vi "processesAbsorptionImage.vi"(8 "error in (no error)":errorcluster, 9 "FileNeologist.lvclass out":refnum<class "FileNeologist.lvclass">, 10 "ImagePaths in":path[](array[path])) -> (0 "error out":errorcluster, 1 "atomNumber":dbl, 2 "ImagePaths out":path[](array[path]), 3 "BECImageProcessor out":refnum<class "BECImageProcessor.lvclass">, 4 "cloudWidth x":dbl, 5 "cloudWidth z":dbl)   [LabVIEW 2009, in "Tools.lvlib" / "Imaging.lvlib" / "BECImageProcessor.lvclass"]
uses:
  BECImageProcessor.lvclass
  Filing/FileNeologist/FileNeologist.lvclass
  <vilib>/vision/NI_Vision_Development_Module.lvlib
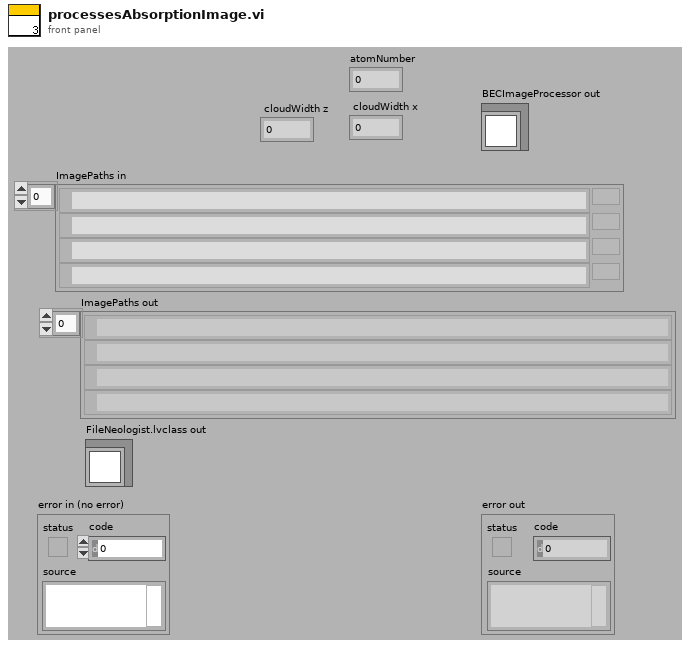
[diagram p1: front panel]
types:
  T1 = typedef "Image Type" = u32
  T2 = typedef "IMAQ Image.ctl" = refnum<image>
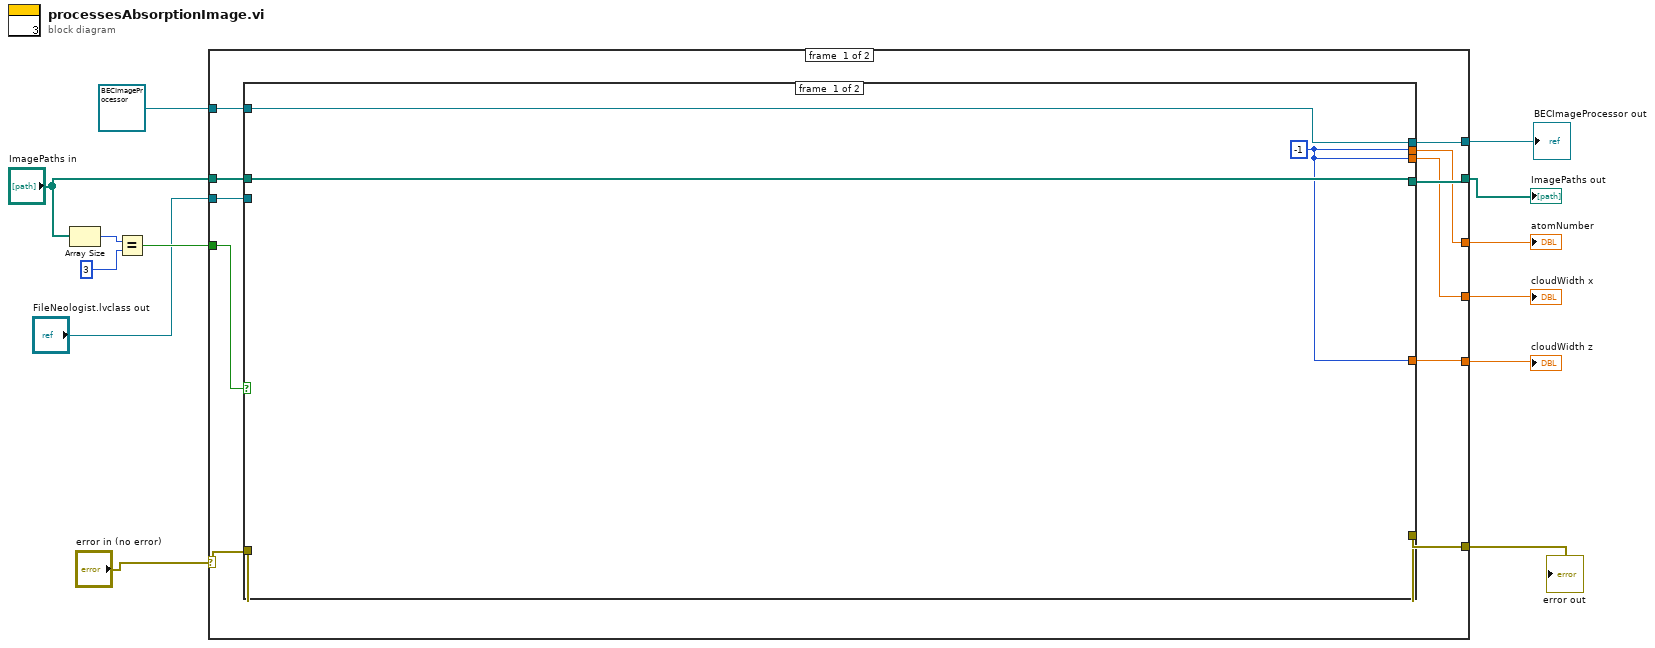
[diagram p0: block diagram]
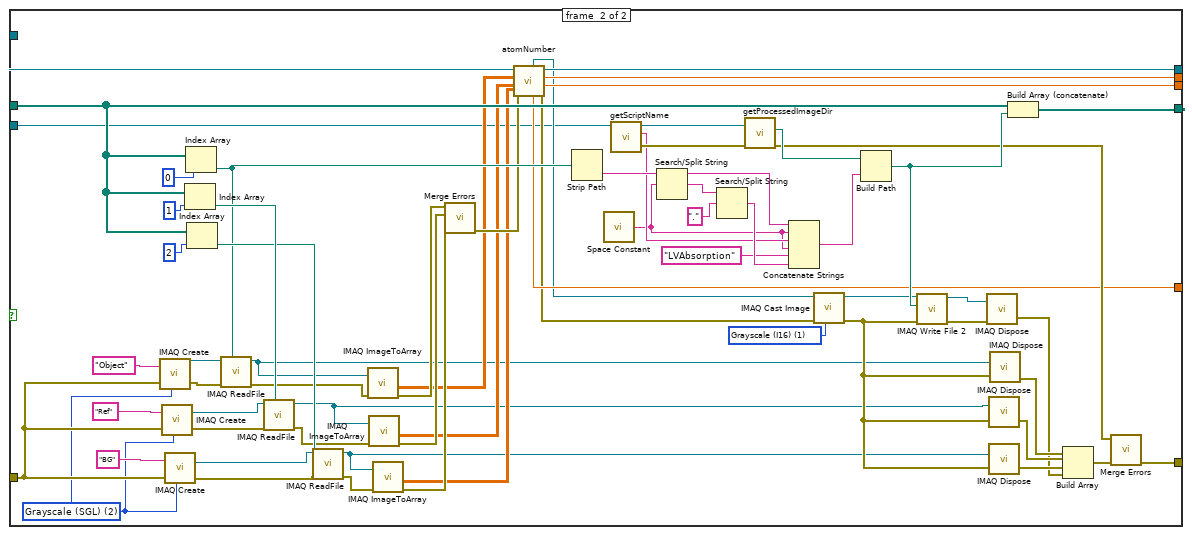
[diagram p2: hidden frame]
diagram:
  n1 = Array Size(array="ImagePaths in") -> (size(s)=w7:i32)
  n2 = Equal?(x=w7, y=3) -> (x = y?=w5:bool)
  n3 = case shown="No Error" "error in (no error)" {
    selector: "error in (no error)" -> [w24 w95]
    tunnel: [w21 w95] -> w10
    tunnel: [w18 w94] -> w12
    tunnel: refnum<class "BECImageProcessor.lvclass"> refnum ("BECImageProcessor in") -> [w19 w94]
    tunnel: "ImagePaths in" -> [w23 _]
    tunnel: [w22 _] -> w11
    tunnel: w5 -> [w20 _]
    tunnel: [w17 _] -> w4
    tunnel: [w16 _] -> w3
    tunnel: [w15 _] -> w2
    tunnel: "FileNeologist.lvclass out" -> [w14 _]
    frame #0 {
      n4 = case shown="True" w20 {
        tunnel: w24 -> [w27 w86]
        tunnel: w23 -> [w28 w78]
        tunnel: [w28 w77] -> w22
        tunnel: [w27 w68] -> w21
        tunnel: w19 -> [w26 w46]
        tunnel: [w26 w41] -> w18
        tunnel: [w25 w40] -> w17
        tunnel: [w25 w39] -> w16
        tunnel: [w25 w38] -> w15
        tunnel: w14 -> [_ w29]
        frame #0 {
          w25 = -1
        }
        frame #1 {
          w60 = T1 1 items=["Grayscale (U8)", "Grayscale (I16)", "Grayscale (SGL)", "Complex (CSG)", "RGB (U32)", "HSL (U32)", "RGB (U64)"] ("Image Type")
          w50 = T1 2 items=["Grayscale (U8)", "Grayscale (I16)", "Grayscale (SGL)", "Complex (CSG)", "RGB (U32)", "HSL (U32)", "RGB (U64)"] ("Image Type")
          n5 = call "IMAQ Create"("Image Name"="Object", "Image Type"=w50, "error in (no error)"=w86) -> ("New Image"=w62:T2, "error out"=w67:errorcluster)  [unwired: 2 in]
          n6 = call "IMAQ Create"("Image Name"="Ref", "Image Type"=w50, "error in (no error)"=w86) -> ("New Image"=w66:T2, "error out"=w65:errorcluster)  [unwired: 2 in]
          n7 = call "IMAQ Create"("Image Name"="BG", "Image Type"=w50, "error in (no error)"=w86) -> ("New Image"=w64:T2, "error out"=w63:errorcluster)  [unwired: 2 in]
          n8 = Index Array(array=w78, index=1) -> (element=w88:path)
          n9 = Index Array(array=w78, index=0) -> (element=w85:path)
          n10 = Index Array(array=w78, index=2) -> (element=w87:path)
          n11 = call "IMAQ ReadFile"("File Path"=w85, "error in (no error)"=w67, "Image"=w62) -> ("error out"=w37:errorcluster, "Image Out"=w34:T2)  [unwired: 4 in, 3 out]
          n12 = call "IMAQ ReadFile"("File Path"=w88, "error in (no error)"=w65, "Image"=w66) -> ("error out"=w36:errorcluster, "Image Out"=w33:T2)  [unwired: 4 in, 3 out]
          n13 = call "IMAQ ReadFile"("File Path"=w87, "error in (no error)"=w63, "Image"=w64) -> ("error out"=w35:errorcluster, "Image Out"=w32:T2)  [unwired: 4 in, 3 out]
          n14 = call "IMAQ ImageToArray"("error in (no error)"=w37, "Image"=w34) -> ("Image Pixels (Float)"=w44:sgl[][], "error out"=w49:errorcluster)  [unwired: 2 in, 3 out]
          n15 = call "IMAQ ImageToArray"("error in (no error)"=w36, "Image"=w33) -> ("Image Pixels (Float)"=w43:sgl[][], "error out"=w48:errorcluster)  [unwired: 2 in, 3 out]
          n16 = call "IMAQ ImageToArray"("error in (no error)"=w35, "Image"=w32) -> ("Image Pixels (Float)"=w42:sgl[][], "error out"=w47:errorcluster)  [unwired: 2 in, 3 out]
          n17 = call <vilib>:"Merge Errors.vi"("error in 3 (no error)"=w47, "error in 2 (no error)"=w48, "error in 1 (no error)"=w49) -> ("error out"=w45:errorcluster)  [unwired: 4 in]
          n18 = call "atomNumber.vi"("Image bg"=w42, "error in (no error)"=w45, "Image ref"=w43, "Image object"=w44, "BECImageProcessor in"=w46) -> ("error out"=w31:errorcluster, "x width"=w39:dbl, "number"=w40:dbl, "BECImageProcessor out"=w41:refnum<class "BECImageProcessor.lvclass">, "z width"=w38:dbl, "Image Out"=w30:T2)  [unwired: 1 in]
          n19 = Strip Path(path=w85) -> (name=w83:string)  [unwired: 1 out]
          n20 = call <vilib>:"Space Constant.vi"() -> ("String"=w51:string)
          n21 = call-dynamic "getScriptName.vi"("FileNeologist.lvclass in"=w29) -> ("error out"=w54:errorcluster, "scriptName"=w53:string, "FileNeologist.lvclass out"=w55:refnum<class "FileNeologist.lvclass">)  [unwired: 8 in]
          n22 = Search/Split String(string=w83, search string/char (-)=w51) -> (substring before match=w81:string, match + rest of string=w82:string)  [unwired: 1 in, 1 out]
          n23 = Search/Split String(string=w82, search string/char (-)=".") -> (match + rest of string=w80:string)  [unwired: 1 in, 2 out]
          n24 = call-dynamic "getProcessedImageDir.vi"("error in (no error)"=w54, "FileNeologist in"=w55) -> ("error out"=w57:errorcluster, "Path"=w58:path)  [unwired: 7 in, 1 out]
          n25 = Concatenate Strings(w81, w51, w53, w51, "LVAbsorption", w80) -> (w79:string)
          n26 = call "IMAQ Cast Image"("Image Type"=w60, "error in (no error)"=w31, "Image Src"=w30) -> ("error out"=w61:errorcluster, "Image Dst Out"=w59:T2)  [unwired: 7 in]
          n27 = Build Path(base path=w58, name or relative path=w79) -> (appended path=w76:path)
          n28 = call-poly "IMAQ Write File 2"("error in (no error)"=w61, "File Path"=w76, "Image"=w59) -> ("error out"=w74:errorcluster, "Image Out (duplicate)"=w75:T2)  [unwired: 7 in]
          n29 = call "IMAQ Dispose"("Image"=w75, "error in (no error)"=w74) -> ("error out"=w70:errorcluster)  [unwired: 4 in]
          n30 = call "IMAQ Dispose"("Image"=w33, "error in (no error)"=w61) -> ("error out"=w72:errorcluster)  [unwired: 4 in]
          n31 = call "IMAQ Dispose"("Image"=w32, "error in (no error)"=w61) -> ("error out"=w71:errorcluster)  [unwired: 4 in]
          n32 = call "IMAQ Dispose"("Image"=w34, "error in (no error)"=w61) -> ("error out"=w73:errorcluster)  [unwired: 4 in]
          n33 = Build Array (concatenate)(w78, w76) -> (w77:path[])
          n34 = Build Array(w73, w72, w71, w70) -> (w69:errorcluster[])
          n35 = call <vilib>:"Merge Errors.vi"("error array in"=w69, "error in 1 (no error)"=w57) -> ("error out"=w68:errorcluster)  [unwired: 5 in]
        }
      }
    }
    frame #1 {
    }
  }
  "error out" <- w10
  "BECImageProcessor out" <- w12
  "ImagePaths out" <- w11
  "atomNumber" <- w4
  "cloudWidth x" <- w3
  "cloudWidth z" <- w2
